vi "Read Topic Info.vi"(11 "Topic in":refnum<class "Topic.lvclass">) -> (2 "Name":string, 3 "Type":string)   [LabVIEW 2015, in "Mediator.lvlib" / "Topic.lvclass"]
uses:
  Topic.lvclass
  Topic.lvclass/Topic.ctl
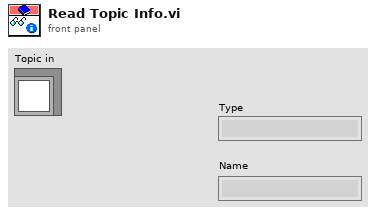
[diagram p1: front panel]
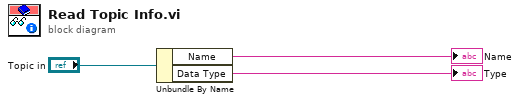
[diagram p0: block diagram]
diagram:
  n1 = Unbundle By Name("Topic in") -> ("Name"=→"Name":string, "Data Type"=→"Type":string)
